vi "HW_7p1_Task2_PRADHASK.vi"() -> ()   [LabVIEW 2016]
panel:
  out "Factorial":dbl
  in  "N":i8
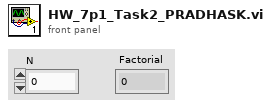
[diagram p1: front panel]
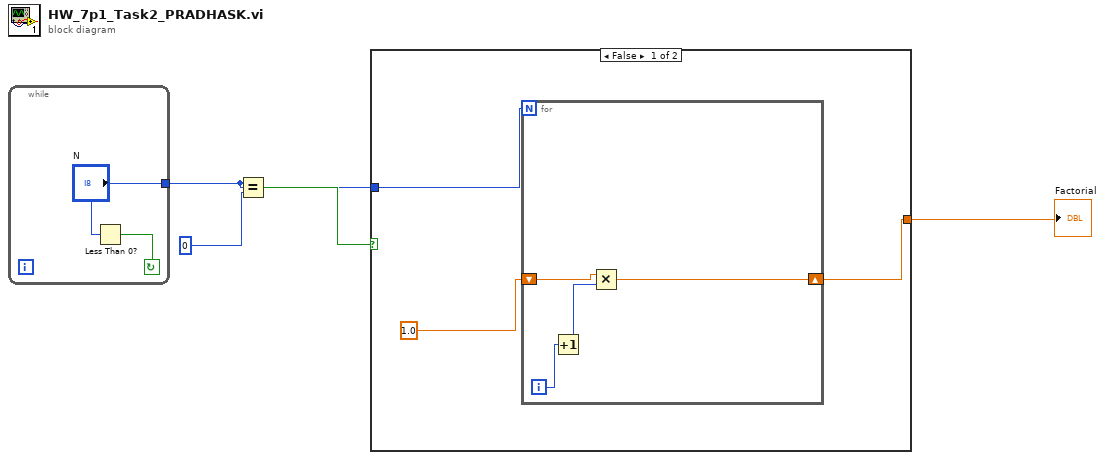
[diagram p0: block diagram]
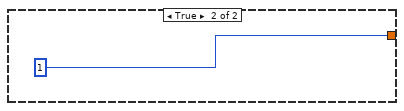
[diagram p2: hidden frame]
diagram:
  n1 = while {
    tunnel: ["N"] -> w1
    stop <- w5 continue-if-true
    n2 = Less Than 0?(x="N") -> (x < 0?=w5:bool)
  }
  n3 = Equal?(x=w1, y=0) -> (x = y?=w3:bool)
  n4 = case shown="False" w3 {
    tunnel: [w7 1] -> w2
    tunnel: w1 -> [w9 _]
    frame False {
      n5 = for {
        N: w9 -> [_]
        shift-right: [w10] -> w7
        shift-left: 1.0 -> [w11]
        i -> [w13]
        n6 = Increment(x=w13) -> (x+1=w12:i32)
        n7 = Multiply(x=w11, y=w12) -> (x*y=w10:dbl)
      }
    }
    frame True {
    }
  }
  "Factorial" <- w2
